vi "Read Variables Egauge.vi"(8 "error in (no error)":errorcluster, 11 "Modbus master in":refnum<class "Modbus Master.lvclass">) -> (0 "error out":errorcluster, 2 "Variables":sgl[](array[numeric]), 3 "Modbus master out":refnum<class "Modbus Master.lvclass">)   [LabVIEW 2019]
uses:
  <vilib>/Modbus/master/Modbus Master.lvclass
panel:
  out "Average AC current":sgl
  out "Phase C current":sgl
  out "Phase B current":sgl
  out "Phase A current":sgl
  out "Power Egauge":sgl
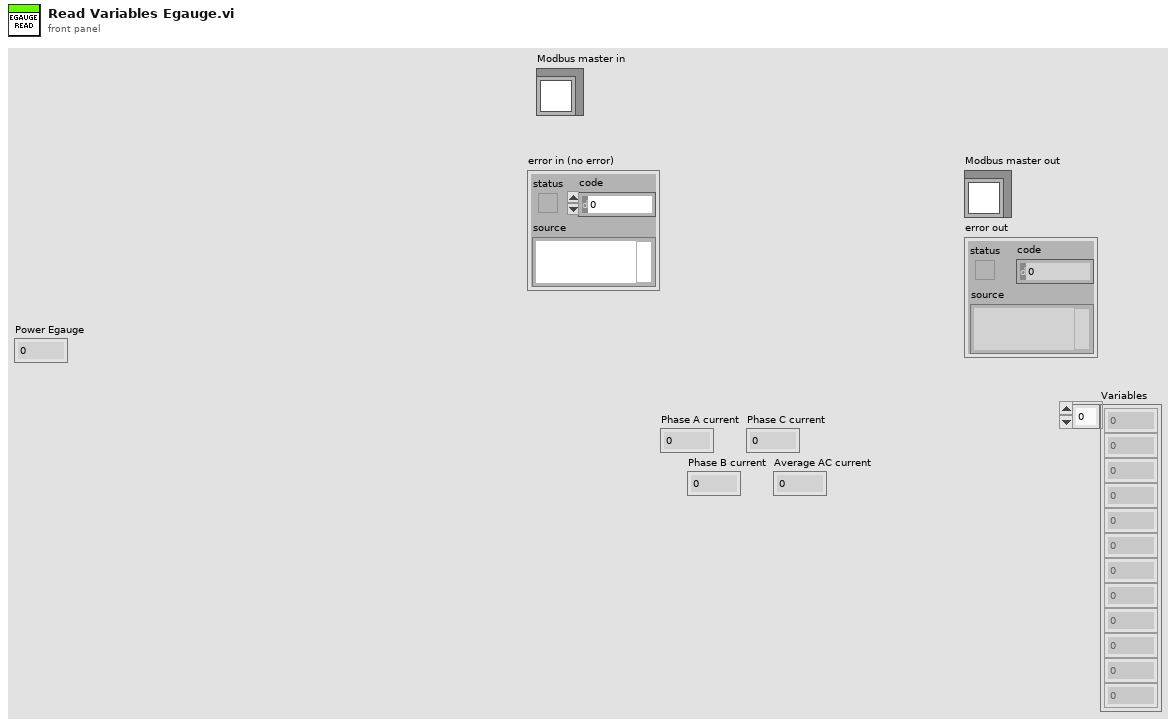
[diagram p1: front panel]
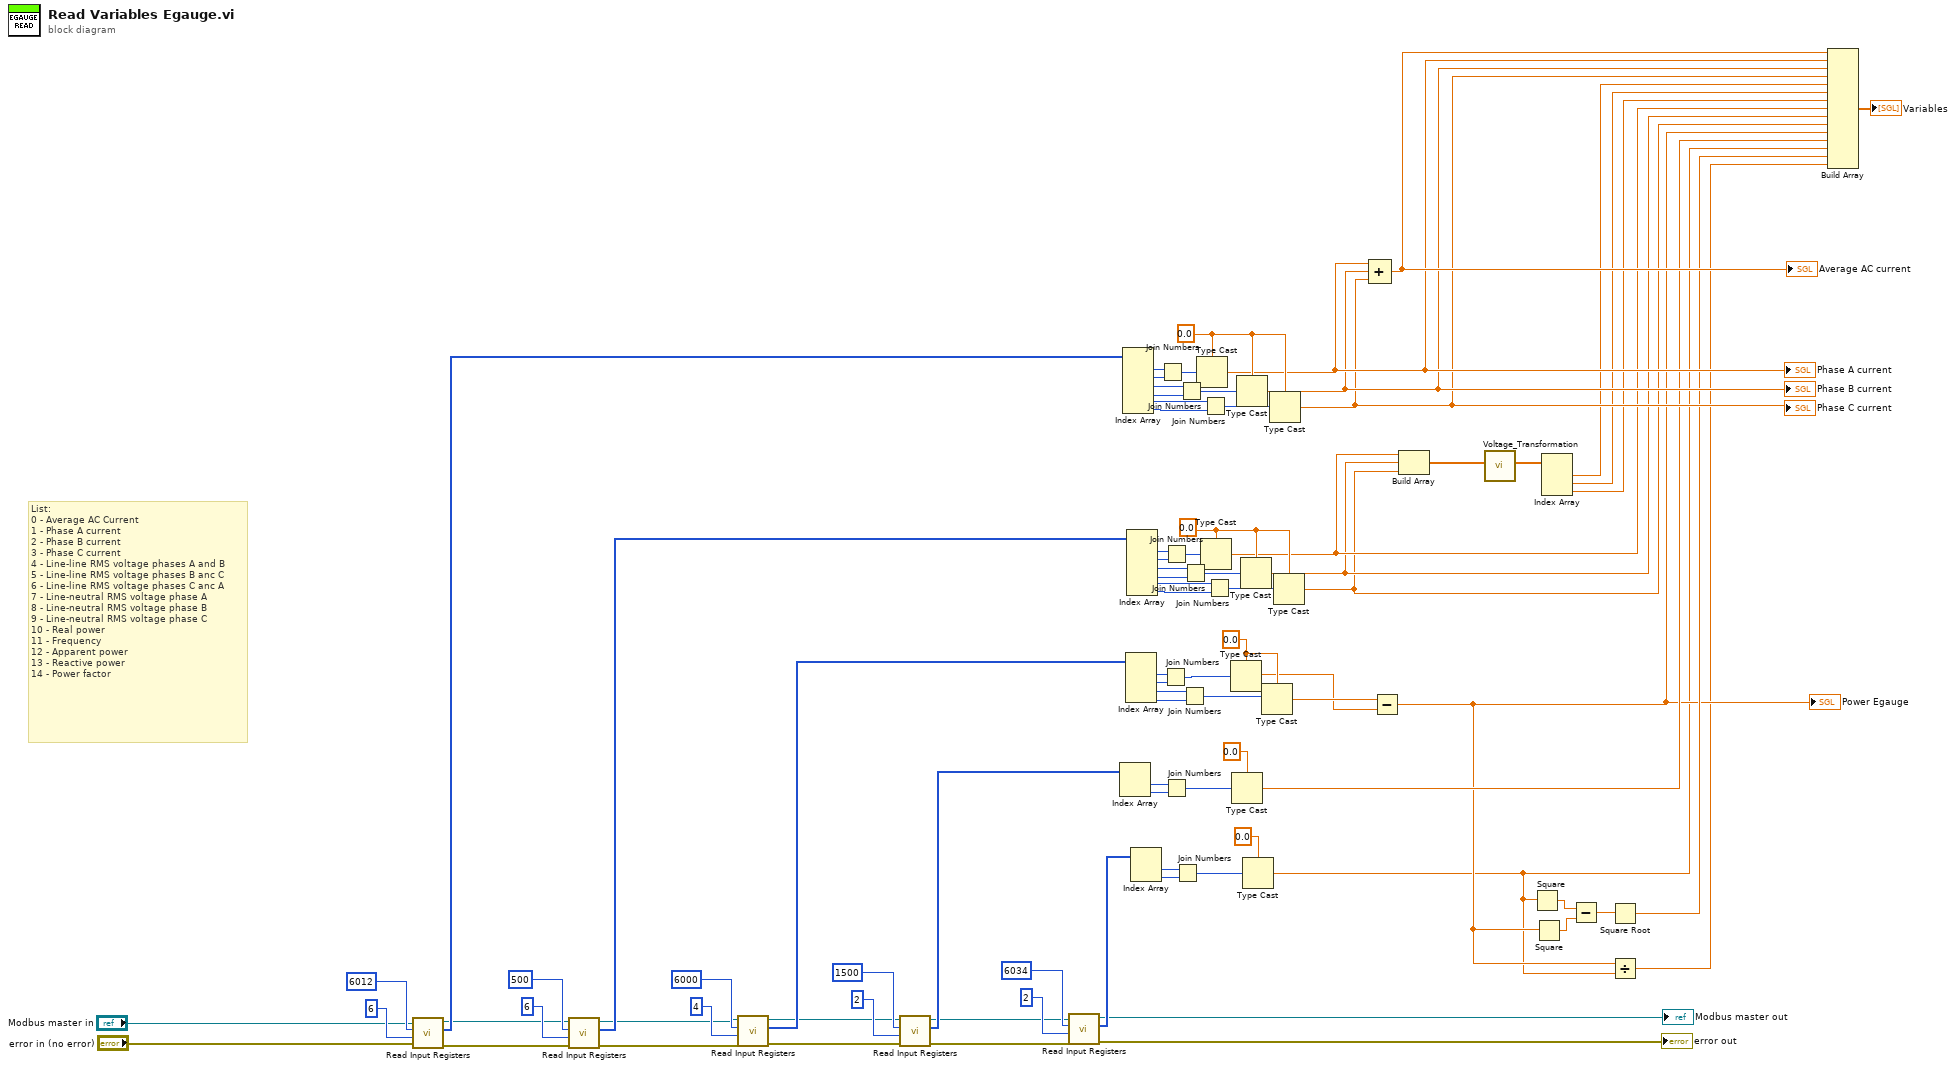
[diagram p0: block diagram]
diagram:
  w47 = sgl 0.0
  w61 = sgl 0.0
  w76 = sgl 0.0
  # "List:\n0 - Average AC Current\n1 - Phase A current\n2 - Phase B current\n3 - Phase C current\n4 - Line-line RMS voltage phases A and B\n5 - Line-line RMS voltage phases B anc C\n6 - Line-line RMS voltage phases C anc A\n7 - Line-neutral RMS voltage phase A\n8 - Line-neutral RMS voltage phase B\n9 - Line-neutral RMS voltage phase C\n10 - Real power\n11 - Frequency\n12 - Apparent power\n13 - Reactive power\n14 - Power factor"
  n1 = call-dynamic "Read Input Registers.vi"("error in (no error)"="error in (no error)", "number of input registers"=u16 6 ("starting address"), "starting address"=u16 6012, "Modbus master in"="Modbus master in") -> ("error out"=w44:errorcluster, "register values"=w46:u16[], "Modbus master out"=w45:refnum<class "Modbus Master.lvclass">)  [unwired: 5 in]
  n2 = call-dynamic "Read Input Registers.vi"("error in (no error)"=w44, "number of input registers"=u16 6 ("starting address"), "starting address"=u16 500, "Modbus master in"=w45) -> ("error out"=w28:errorcluster, "register values"=w65:u16[], "Modbus master out"=w29:refnum<class "Modbus Master.lvclass">)  [unwired: 5 in]
  n3 = call-dynamic "Read Input Registers.vi"("error in (no error)"=w28, "number of input registers"=u16 4 ("starting address"), "starting address"=u16 6000, "Modbus master in"=w29) -> ("error out"=w27:errorcluster, "register values"=w83:u16[], "Modbus master out"=w26:refnum<class "Modbus Master.lvclass">)  [unwired: 5 in]
  n4 = call-dynamic "Read Input Registers.vi"("error in (no error)"=w27, "number of input registers"=u16 2 ("starting address"), "starting address"=u16 1500, "Modbus master in"=w26) -> ("error out"=w16:errorcluster, "register values"=w25:u16[], "Modbus master out"=w17:refnum<class "Modbus Master.lvclass">)  [unwired: 5 in]
  n5 = call-dynamic "Read Input Registers.vi"("error in (no error)"=w16, "number of input registers"=u16 2 ("starting address"), "starting address"=u16 6034, "Modbus master in"=w17) -> ("error out"=→"error out":errorcluster, "register values"=w11:u16[], "Modbus master out"=→"Modbus master out":refnum<class "Modbus Master.lvclass">)  [unwired: 5 in]
  n6 = Index Array(array=w25) -> (element #1=w22:u16, element #2=w21:u16)  [unwired: 2 in]
  n7 = Index Array(array=w46) -> (element #1=w56:u16, element #2=w55:u16, element #3=w53:u16, element #4=w52:u16, element #5=w50:u16, element #6=w49:u16)  [unwired: 6 in]
  n8 = Index Array(array=w83) -> (element #1=w82:u16, element #2=w81:u16, element #3=w79:u16, element #4=w78:u16)  [unwired: 4 in]
  n9 = Index Array(array=w65) -> (element #1=w71:u16, element #2=w70:u16, element #3=w68:u16, element #4=w67:u16, element #5=w64:u16, element #6=w63:u16)  [unwired: 6 in]
  n10 = Index Array(array=w11) -> (element #1=w13:u16, element #2=w12:u16)  [unwired: 2 in]
  n11 = Join Numbers(hi=w56, lo=w55) -> ((hi.lo)=w54:u32)
  n12 = Join Numbers(hi=w82, lo=w81) -> ((hi.lo)=w80:u32)
  n13 = Join Numbers(hi=w71, lo=w70) -> ((hi.lo)=w69:u32)
  n14 = Join Numbers(hi=w22, lo=w21) -> ((hi.lo)=w24:u32)
  n15 = Join Numbers(hi=w13, lo=w12) -> ((hi.lo)=w15:u32)
  n16 = Join Numbers(hi=w53, lo=w52) -> ((hi.lo)=w51:u32)
  n17 = Join Numbers(hi=w79, lo=w78) -> ((hi.lo)=w77:u32)
  n18 = Join Numbers(hi=w68, lo=w67) -> ((hi.lo)=w66:u32)
  n19 = Type Cast(type=w47, x=w54) -> (*(type *) &x=w39:sgl)
  "Phase A current" <- w39
  n20 = Join Numbers(hi=w50, lo=w49) -> ((hi.lo)=w48:u32)
  n21 = Type Cast(type=w61, x=w69) -> (*(type *) &x=w32:sgl)
  n22 = Join Numbers(hi=w64, lo=w63) -> ((hi.lo)=w62:u32)
  n23 = Type Cast(type=w76, x=w80) -> (*(type *) &x=w74:sgl)
  n24 = Type Cast(type=sgl 0.0, x=w24) -> (*(type *) &x=w20:sgl)
  n25 = Type Cast(type=w47, x=w51) -> (*(type *) &x=w38:sgl)
  "Phase B current" <- w38
  n26 = Type Cast(type=w61, x=w66) -> (*(type *) &x=w31:sgl)
  n27 = Type Cast(type=sgl 0.0, x=w15) -> (*(type *) &x=w5:sgl)
  n28 = Type Cast(type=w76, x=w77) -> (*(type *) &x=w75:sgl)
  n29 = Type Cast(type=w47, x=w48) -> (*(type *) &x=w37:sgl)
  "Phase C current" <- w37
  n30 = Type Cast(type=w61, x=w62) -> (*(type *) &x=w30:sgl)
  n31 = Compound Arithmetic op=ADD(w39, w38, w37) -> (w40:sgl)
  "Average AC current" <- w40
  n32 = Subtract(x=w75, y=w74) -> (x-y=w6:sgl)
  "Power Egauge" <- w6
  n33 = Build Array(w32, w31, w30) -> (w43:sgl[])
  n34 = call "Voltage_Transformation.vi"("VLL"=w43) -> ("VLN"=w36:sgl[])  [unwired: 10 in]
  n35 = Square(x=w5) -> (x^2=w10:sgl)
  n36 = Square(x=w6) -> (x^2=w9:sgl)
  n37 = Index Array(array=w36) -> (element #1=w35:sgl, element #2=w34:sgl, element #3=w33:sgl)  [unwired: 3 in]
  n38 = Subtract(x=w10, y=w9) -> (x-y=w8:sgl)
  n39 = Square Root(x=w8) -> (sqrt(x)=w7:sgl)
  n40 = Divide(x=w6, y=w5) -> (x/y=w4:sgl)
  n41 = Build Array(w40, w39, w38, w37, w35, w34, w33, w32, w31, w30, w6, w20, w5, w7, w4) -> (→"Variables":sgl[])
